vi "SAC-Create Stimulus.vi"(0 "Params":T1={"Fs (Hz)"=0.0, "atten (dB)"=0.0, "Waveform"=enum."Chirp", "Freq Res (Hz)"=0.0, "Order"=0, "Averages"=0, "seed"=-1, "Window"={"Type"=enum."None", "Length (ms)"=0.0, "Center (ms)"=0.0}, "Mic gain"=0.0, "Mic sens"=0.0}) -> (3 "duration (ms)":dbl, 4 "Stimulus":dbl[](array[numeric]), 6 "time":cluster{i32, "dx":dbl, "Y":dbl[]}, 8 "autocorr":cluster{dbl, "dx":dbl, "Y":dbl[]}, 10 "mag":cluster{i32, "dx":dbl, "Y":dbl[]}, 15 "phase":cluster{i32, "dx":dbl, "Y":dbl[]})   [LabVIEW 2020]
uses:
  Typedefs/SAC-Parameters.ctl
  HRTF VIs/Typedefs/HRTF-Waveform.ctl
  HRTF VIs/Typedefs/HRTF-Window.ctl
  HRTF VIs/Typedefs/HRTF-Window Type.ctl
  EPhys/LV Source/Calibration VIs/Typedefs/ACal-Stimulus Properties.ctl
  <vilib>/Analysis/2dsp.llb/1D Auto Correlation (DBL).vi
  Utility VIs/Math VIs/dB to Linear (scalar).vi
  Utility VIs/Math VIs/FFT x(t) to dB,Degrees (1D).vi
  <vilib>/Analysis/NI_AALBase.lvlib
  <vilib>/Analysis/NI_AALPro.lvlib
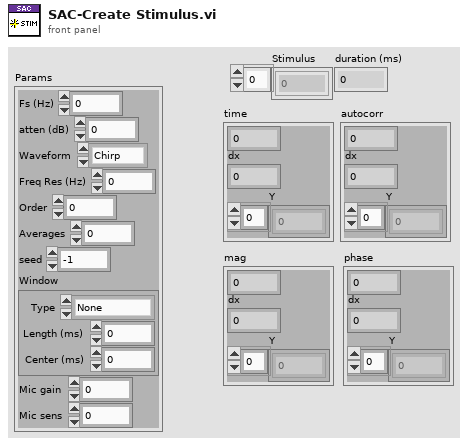
[diagram p1: front panel]
types:
  T1 = typedef "SAC-Parameters.ctl" = cluster{"Fs (Hz)":dbl, "atten (dB)":dbl, "Waveform":T2, "Freq Res (Hz)":dbl, "Order":i32, "Averages":i32, "seed":i64, "Window":T3, "Mic gain":dbl, "Mic sens":dbl}
  T2 = typedef "HRTF-Waveform.ctl" = enum16{"Chirp", "MLS"}
  T3 = typedef "HRTF-Window.ctl" = cluster{"Type":T4, "Length (ms)":dbl, "Center (ms)":dbl}
  T4 = typedef "HRTF-Window Type.ctl" = enum16{"None", "Rectangle", "Hanning"}
  T5 = typedef "ACal-Stimulus Properties.ctl" = cluster{"Freq Step (Hz)":dbl, "Waveform":enum16{"Chirp"}, "Attenuation (dB)":dbl, "Sample Rate (Hz)":dbl, "Fmin (Hz)":dbl, "Fmax (Hz)":dbl}
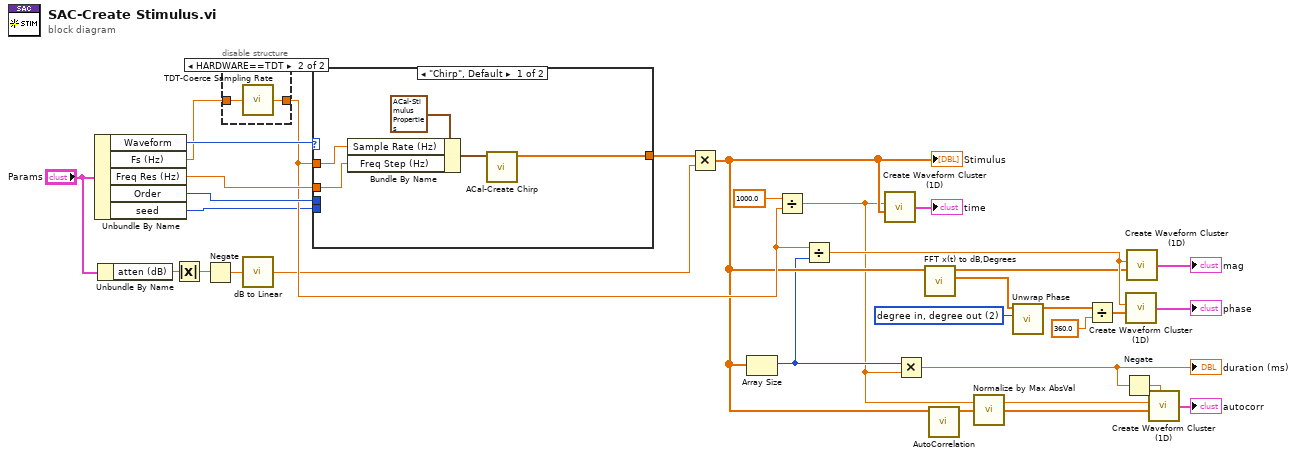
[diagram p0: block diagram]
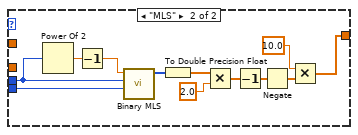
[diagram p3: hidden frame]
diagram:
  w9 = 2 items=["radian in, radian out", "radian in, degree out", "degree in, degree out", "degree in, radian out"] ("phase unit")
  n1 = Unbundle By Name("Params") -> ("Waveform"=w31:T2, "Fs (Hz)"=w29:dbl, "Freq Res (Hz)"=w30:dbl, "Order"=w26:i32, "seed"=w1:i64)
  n2 = Unbundle By Name("Params") -> ("atten (dB)"=w3:dbl)
  n3 = Absolute Value(x=w3) -> (abs(x)=w21:dbl)
  n4 = Negate(x=w21) -> (-x=w20:dbl)
  n5 = disable-structure shown="HARDWARE==TDT" {
    disable-tunnel: w29 -> [w32 w34]
    disable-tunnel: [w32 w33] -> w22
    frame condition #0 {
    }
    frame condition #1 (active) {
      n6 = call "TDT-Coerce Sampling Rate.vi"("Fs (Hz)"=w34) -> ("Coerced"=w33:dbl)
    }
  }
  n7 = call-poly "dB to Linear.vi"("dB"=w20) -> ("linear"=w19:dbl)
  n8 = case shown="\"Chirp\", Default" w31 {
    tunnel: w30 -> [w39 _]
    tunnel: w22 -> [w38 _]
    tunnel: [w35 w42] -> w23
    tunnel: w26 -> [_ w51]
    tunnel: w1 -> [_ w40]
    frame "Chirp", Default {
      n9 = Bundle By Name(cluster=T5 {"Freq Step (Hz)"=50.0, "Waveform"=enum."Chirp", "Attenuation (dB)"=50.0, "Sample Rate (Hz)"=0.0, "Fmin (Hz)"=20.0, "Fmax (Hz)"=100000.0} ("Cal.Stimulus"), "Sample Rate (Hz)"=w38, "Freq Step (Hz)"=w39) -> (w36:T5)
      n10 = call "ACal-Create Chirp.vi"("Cal.Stimulus"=w36) -> ("Stimulus"=w35:dbl[])  [unwired: 9 in, 1 out]
    }
    frame "MLS" {
      n11 = Power Of 2(x=w51) -> (2^x=w50:dbl)
      n12 = Decrement(x=w50) -> (x-1=w49:dbl)
      n13 = call <vilib>:"Binary MLS.vi"("seed"=w40, "polynomial order"=w51, "samples"=w49) -> ("mls sequence"=w48:u8[])  [unwired: 7 in, 1 out]
      n14 = To Double Precision Float(number=w48) -> (double precision float=w44:dbl[])
      n15 = Multiply(x=w44, y=2.0) -> (x*y=w46:dbl[])
      n16 = Decrement(x=w46) -> (x-1=w43:dbl[])
      n17 = Negate(x=w43) -> (-x=w45:dbl[])
      n18 = Multiply(x=10.0, y=w45) -> (x*y=w42:dbl[])
    }
  }
  n19 = Multiply(x=w23, y=w19) -> (x*y=w18:dbl[])
  "Stimulus" <- w18
  n20 = Array Size(array=w18) -> (size(s)=w13:i32)
  n21 = Divide(x=1000.0, y=w22) -> (x/y=w4:dbl)
  n22 = Divide(x=w22, y=w13) -> (x/y=w15:dbl)
  n23 = call "Create Waveform Cluster (1D).vi"("dx"=w4, "Y"=w18) -> ("waveform cluster"=→"time":cluster{dbl, "dx":dbl, "Y":dbl[]})  [unwired: 3 in]
  n24 = Multiply(x=w13, y=w4) -> (x*y=w2:dbl)
  "duration (ms)" <- w2
  n25 = call-poly "FFT x(t) to dB,Degrees.vi"("X"=w18) -> ("+Freq Phase of FFT (degrees)"=w7:dbl[], "+Freq. Mag of FFT (dB rms)"=w8:dbl[])  [unwired: 8 in, 1 out]
  n26 = call-poly <vilib>:"AutoCorrelation.vi"("X"=w18) -> ("Rxx"=w11:dbl[])  [unwired: 9 in, 1 out]
  n27 = call "Normalize by Max AbsVal.vi"("Y"=w11) -> ("Ynorm"=w12:dbl[])
  n28 = call <vilib>:"Unwrap Phase.vi"("phase unit"=w9, "Phase"=w7) -> ("Unwrapped Phase"=w6:dbl[])  [unwired: 8 in, 1 out]
  n29 = Divide(x=w6, y=360.0) -> (x/y=w16:dbl[])
  n30 = Negate(x=w2) -> (-x=w10:dbl)
  n31 = call "Create Waveform Cluster (1D).vi"("dx"=w15, "Y"=w16) -> ("waveform cluster"=→"phase":cluster{dbl, "dx":dbl, "Y":dbl[]})  [unwired: 3 in]
  n32 = call "Create Waveform Cluster (1D).vi"("dx"=w15, "Y"=w8) -> ("waveform cluster"=→"mag":cluster{dbl, "dx":dbl, "Y":dbl[]})  [unwired: 3 in]
  n33 = call "Create Waveform Cluster (1D).vi"("dx"=w4, "Y"=w12, "offset"=w10) -> ("waveform cluster"=→"autocorr":cluster{dbl, "dx":dbl, "Y":dbl[]})  [unwired: 2 in]
